vi "libssh2_session_set_blocking - invalid session - no error 1097.vi"() -> ()   [LabVIEW 2013, in "libssh2_tests.lvlib"]
uses:
  libssh2/Session Refnum.ctl
  libssh2/libssh2_init_default.vi
  <vilib>/addons/_JKI Toolkits/Caraya/classes/Assert/Assert Not Equal Value_Variant.vi
  libssh2_tests.lvlib
  <vilib>/addons/_JKI Toolkits/Caraya/classes/Test/Test.lvclass
  libssh2/libssh2.lvlib
  <vilib>/addons/_JKI Toolkits/Caraya/classes/Assert/Assert.lvclass
panel:
  out "error out":errorcluster
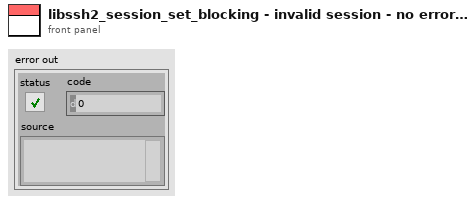
[diagram p1: front panel]
types:
  T1 = typedef "libssh2.lvlib/Session Refnum.ctl" = refnum<k1>
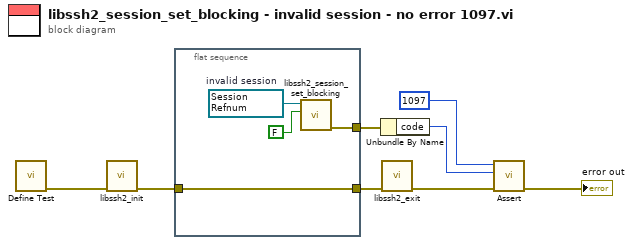
[diagram p0: block diagram]
diagram:
  n1 = call <vilib>:"Define Test.vi"() -> ("error out"=w7:errorcluster)  [unwired: 10 in, 1 out]
  n2 = call-poly "libssh2_init.vi"("error in (no error)"=w7) -> ("error out"=w4:errorcluster)  [unwired: 10 in]
  n3 = flat-sequence {
    tunnel: [w11] -> w5
    tunnel: w4 -> [w11]
    tunnel: [w10] -> w3
    frame #0 {
      w12 = T1 refnum items=["Session"]  # invalid session
      n4 = call "libssh2_session_set_blocking.vi"("blocking"=FALSE, "session"=w12) -> ("error out"=w10:errorcluster)  [unwired: 9 in]
    }
  }
  n5 = Unbundle By Name(w3) -> ("code"=w2:i32)
  n6 = call "libssh2_exit.vi"("error in (no error)"=w5) -> ("error out"=w6:errorcluster)  [unwired: 10 in]
  n7 = call-poly <vilib>:"Assert.vi"("error in (no error)"=w6, "Y"=w2, "X"=1097 ("code")) -> ("error out"=→"error out":errorcluster)  [unwired: 7 in, 1 out]
